vi "Remove.vi"(8 "error in (no error)":errorcluster, 10 "Index":i32, 11 "List in":refnum<class "List.lvclass">) -> (0 "error out":errorcluster, 1 "Item":refnum<class>, 3 "List out":refnum<class "List.lvclass">)   [LabVIEW 2017, in "LapDog.Collections.v0.Lists.lvlib" / "List.lvclass"]
doc: "Removes an item from the list at the given Index. An Index of -1 removes the last item in the list. If no item exists at the given Index error 510301 is returned."
uses:
  List.lvclass
  List.lvclass/List.ctl
  ListImp/ListImp.lvclass
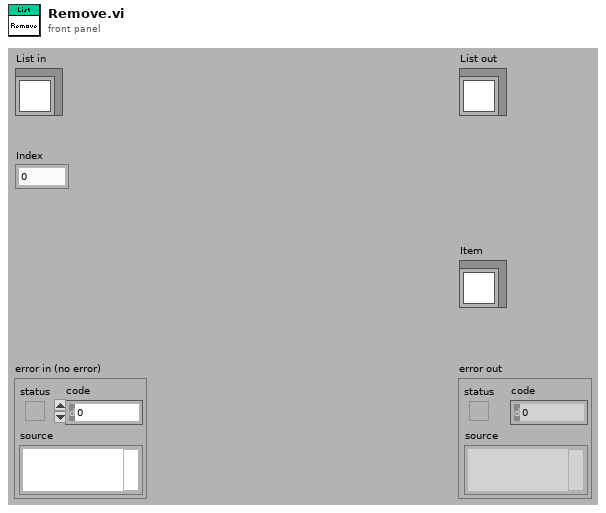
[diagram p1: front panel]
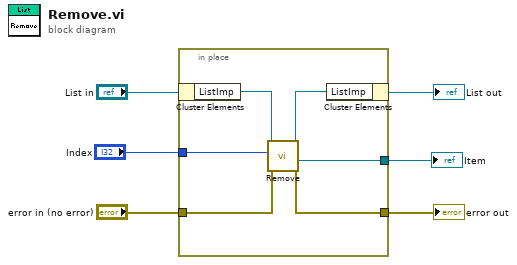
[diagram p0: block diagram]
diagram:
  n1 = in-place {
    in-place-border: "error in (no error)" -> [w12]
    in-place-border: [w11] -> w1
    in-place-border: "Index" -> [w10]
    in-place-border: [w9] -> w3
    n2 = in-place-cluster #1("List in") -> ("ListImp"=w8:refnum<class "ListImp.lvclass">)
    n3 = call-dynamic "Remove.vi"("error in (no error)"=w12, "Index"=w10, "ListImp in"=w8) -> ("error out"=w11:errorcluster, "Item"=w9:refnum<class>, "ListImp out"=w7:refnum<class "ListImp.lvclass">)  [unwired: 6 in]
    n4 = in-place-cluster #1("ListImp"=w7) -> (→"List out":refnum<class "List.lvclass">)
  }
  "error out" <- w1
  "Item" <- w3
